vi "SetClassVal_dump.vi"(8 "error in (no error)":errorcluster caption="entrée d'erreur (pas d'erreur)", 11 "Interface en entrée":refnum<class "Interface.lvclass"> caption="DNL_LabVIEW Object in") -> (0 "error out":errorcluster caption="sortie d'erreur", 3 "Interface en sortie":refnum<class "Interface.lvclass"> caption="DNL_LabVIEW Object out")   [LabVIEW 2019]
uses:
  Interface.lvclass
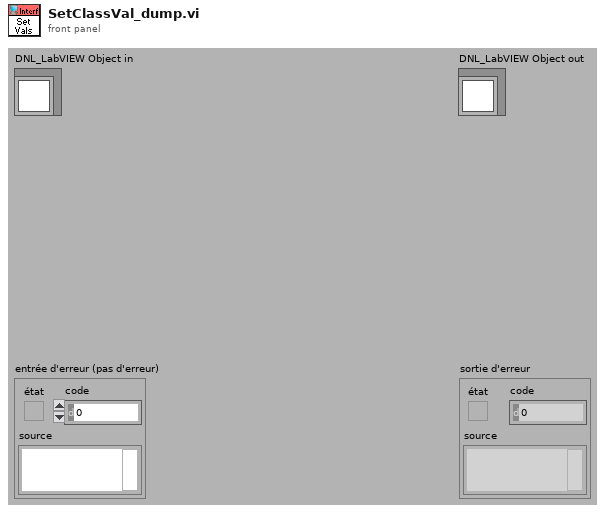
[diagram p1: front panel]
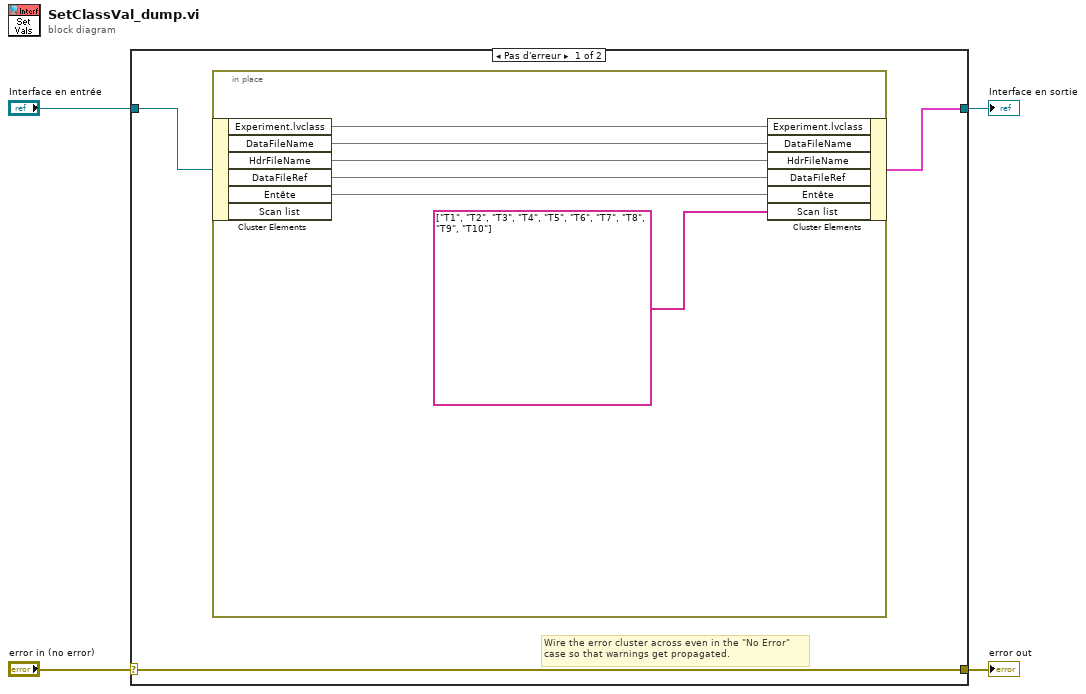
[diagram p0: block diagram]
diagram:
  n1 = case shown="Pas d'erreur" "error in (no error)" {
    selector: "error in (no error)" -> [w7 w15]
    tunnel: [w7 w15] -> w3
    tunnel: [w5 w14] -> w2
    tunnel: "Interface en entrée" -> [w6 w14]
    frame No Error {
      # "Wire the error cluster across even in the \"No Error\"\ncase so that warnings get propagated."
      n2 = in-place {
        n3 = in-place-cluster #1(w6) -> ("Experiment.lvclass"=w13, "DataFileName"=w12, "HdrFileName"=w11, "DataFileRef"=w10, "Entête"=w9)  [unwired: 1 out]
        n4 = in-place-cluster #1("Experiment.lvclass"=w13, "DataFileName"=w12, "HdrFileName"=w11, "DataFileRef"=w10, "Entête"=w9, "Scan list"=string[] ["T1", "T2", "T3", "T4", "T5", "T6", "T7", "T8", "T9", "T10"] ("ScanParams.Scan list")) -> (w5:cluster{})
      }
    }
    frame Error {
    }
  }
  "error out" <- w3
  "Interface en sortie" <- w2
